vi "Measure.vi"(6 "error in (no error)":errorcluster, 9 "Fluke Hydra 2625A in":refnum<class "Fluke Hydra 2625A.lvclass">) -> (0 "error out":errorcluster, 2 "Array of Measurement":dbl[](array[numeric]), 3 "Fluke Hydra 2625A out":refnum<class "Fluke Hydra 2625A.lvclass">)   [LabVIEW 2014, in "Generic Data Acquisition.lvlib" / "Fluke Hydra.lvlib" / "Fluke Hydra 2625A.lvclass"]
uses:
  Fluke Hydra 2625A.lvclass
  <instrlib>/Fluke 2625A/Fluke 2625A.lvlib
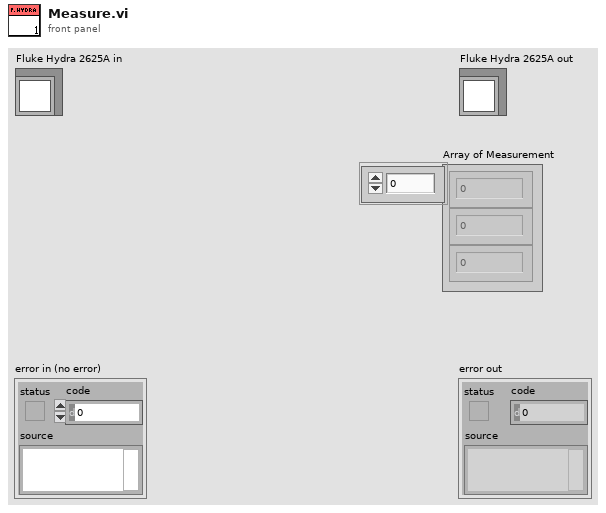
[diagram p1: front panel]
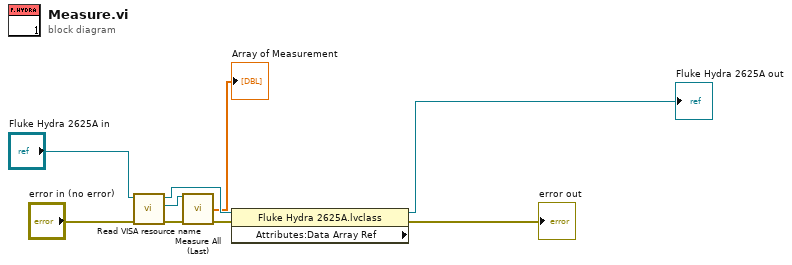
[diagram p0: block diagram]
diagram:
  n1 = call-dynamic "Read VISA resource name.vi"("error in (no error)"="error in (no error)", "Generic Instrument in"="Fluke Hydra 2625A in") -> ("error out"=w6:errorcluster, "VISA resource name"=w8:refnum<visa-resource-name>, "Generic Instrument out"=w5:refnum<class "Fluke Hydra 2625A.lvclass">)  [unwired: 7 in]
  n2 = call <instrlib>:"Measure All (Last).vi"("VISA Resource Name In"=w8, "Error In"=w6) -> ("Numeric Array Out"=→"Array of Measurement":dbl[], "Error Out"=w3:errorcluster)  [unwired: 9 in, 3 out]
  n3 = property class="Fluke Hydra 2625A.lvclass" props=["Attributes:Data Array Ref"](reference=w5, error in=w3) -> (reference out=→"Fluke Hydra 2625A out":refnum<class "Fluke Hydra 2625A.lvclass">, error out=→"error out":errorcluster)  [unwired: 1 out]
